vi "AcquireStartCameraAndReferences.vi"(8 "error in (no error)":errorcluster, 9 "?":T2 {"Image Type" items=["Grayscale (U8)", "Grayscale (I16)", "Grayscale (SGL)", "Complex (CSG)", "RGB (U32)", "HSL (U32)", "RGB (U64)", "Grayscale (U16)"]}, 10 "Settings":T4={"Harware Configuration"={"Camera"="cam1", "Frames Per Second"=15, "Simulate Recording"=FALSE, "Simulated Recording Sample"=path "", "Timestamp Method"=enum."Camera Timestamp"}, "Base Recording Path"=path "", "Type Of Recording"="", "Recording Codec"="", "TrackingSettings"={"Max Radius"=0, "Threshold"=160.0, "ROI"={"Left"=0, "Top"=0, "Right"=0, "Bottom"=0, "Rotation"=0.0}}, "Calibration"={"Pixel Width (X)"=1.0, "Pixel Height (Y)"=1.0}, "Broadcast Length"=0} {"Broadcast Length" min=0; "TrackingSettings"."ROI"."Rotation" format="%.2f"; "TrackingSettings"."ROI"."Left" scale=0.0..1024.0; "TrackingSettings"."ROI"."Right" scale=0.0..1024.0; "TrackingSettings"."Threshold" scale=0.0..255.0}) -> (0 "error out":errorcluster, 1 "?":T2 {"Image Type" items=["Grayscale (U8)", "Grayscale (I16)", "Grayscale (SGL)", "Complex (CSG)", "RGB (U32)", "HSL (U32)", "RGB (U64)", "Grayscale (U16)"]})   [LabVIEW 2017, in "ImageAcquisitionLibrary.lvlib"]
uses:
  ImageAcquisitionLibrary.lvlib
  Settings/Settings.ctl
  <vilib>/userdefined/High Color/IMAQdx.ctl
  Tracking/TrackingSettings.ctl
  Settings/Calibration.ctl
  AcquisitionObject.ctl
  <vilib>/vision/Image Controls.llb/IMAQ Image.ctl
  <vilib>/vision/driver/NI_Vision_Acquisition_Software.lvlib
panel:
  out "Image":T1(plugin-control)
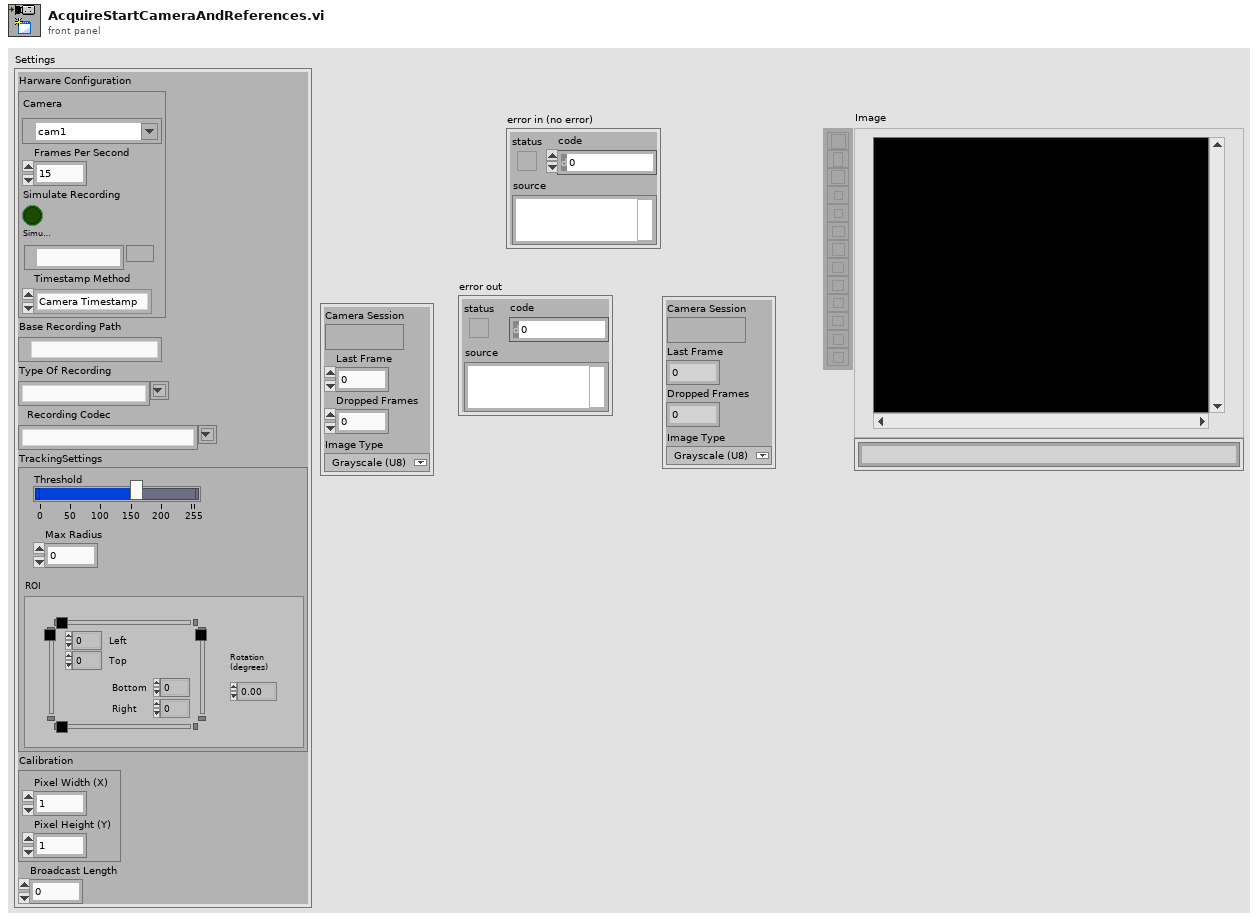
[diagram p1: front panel]
types:
  T1 = typedef "IMAQ Image.ctl" = refnum<image>
  T2 = typedef "ImageAcquisitionLibrary.lvlib/AcquisitionObject.ctl" = cluster{"Camera Session":T1, "Last Frame":u32, "Dropped Frames":u32, "Image Type":T3}
  T3 = typedef "Image Type" = u32
  T4 = typedef "ImageAcquisitionLibrary.lvlib/Settings.ctl" = cluster{"Harware Configuration":cluster{"Camera":T5, "Frames Per Second":u32, "Simulate Recording":bool, "Simulated Recording Sample":path, "Timestamp Method":enum16{"System Timestamp", "Camera Timestamp", "IMAQdx Timestamp"}}, "Base Recording Path":path, "Type Of Recording":string, "Recording Codec":string, "TrackingSettings":T6, "Calibration":T8, "Broadcast Length":i32}
  T5 = typedef "IMAQdx.ctl" = refnum<k21>
  T6 = typedef "ImageAcquisitionLibrary.lvlib/TrackingSettings.ctl" = cluster{"Max Radius":i32, "Threshold":sgl, "ROI":T7}
  T7 = typedef "IMAQ Rectangle" = cluster{"Left":i32, "Top":i32, "Right":i32, "Bottom":i32, "Rotation":dbl}
  T8 = typedef "ImageAcquisitionLibrary.lvlib/Calibration.ctl" = cluster{"Pixel Width (X)":dbl, "Pixel Height (Y)":dbl}
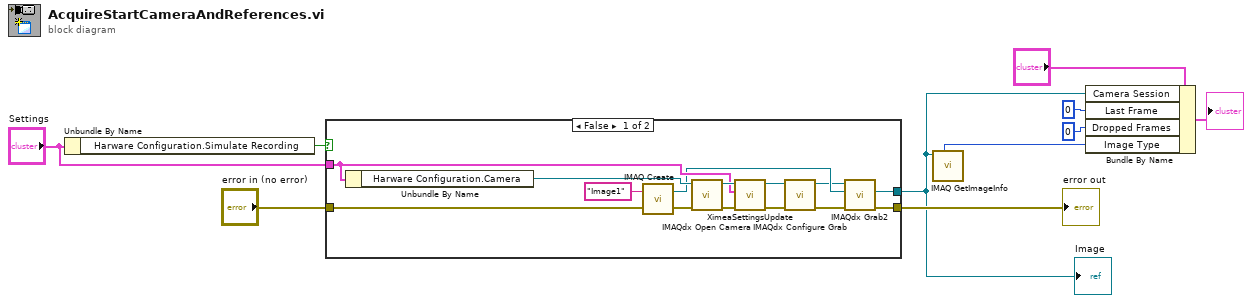
[diagram p0: block diagram]
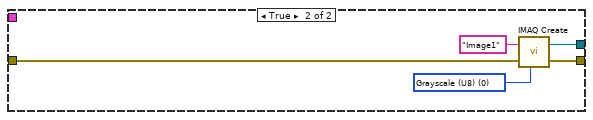
[diagram p2: hidden frame]
diagram:
  n1 = Unbundle By Name("Settings") -> ("Harware Configuration.Simulate Recording"=w9:bool)
  n2 = case shown="False" w9 {
    tunnel: "Settings" -> [w16 _]
    tunnel: "error in (no error)" -> [w23 w27]
    tunnel: [w11 w26] -> w2
    tunnel: [w14 w25] -> w3
    frame False {
      n3 = Unbundle By Name(w16) -> ("Harware Configuration.Camera"=w20:T5)
      n4 = call "IMAQ Create"("Image Name"="Image1", "error in (no error)"=w23) -> ("New Image"=w13:T1, "error out"=w19:errorcluster)  [unwired: 3 in]
      n5 = call <vilib>:"IMAQdx Open Camera.vi"("error in"=w19, "Session In"=w20) -> ("error out"=w21:errorcluster, "Session Out"=w22:T5)  [unwired: 8 in]
      n6 = call "XimeaSettingsUpdate.vi"("error in"=w21, "Cluster"=w16, "Session In"=w22) -> ("error out"=w18:errorcluster, "IMAQdx Session"=w17:T5)  [unwired: 7 in]
      n7 = call <vilib>:"IMAQdx Configure Grab.vi"("error in"=w18, "Session In"=w17) -> ("error out"=w15:errorcluster, "Session Out"=w12:T5)  [unwired: 8 in]
      n8 = call <vilib>:"IMAQdx Grab2.vi"("error in"=w15, "Image In"=w13, "Session In"=w12) -> ("error out"=w14:errorcluster, "Image Out"=w11:T1)  [unwired: 5 in, 2 out]
    }
    frame True {
      w29 = T3 0 items=["Grayscale (U8)", "Grayscale (I16)", "Grayscale (SGL)", "Complex (CSG)", "RGB (U32)", "HSL (U32)", "RGB (U64)", "Grayscale (U16)"] ("Image Type")
      n9 = call "IMAQ Create"("Image Name"="Image1", "Image Type"=w29, "error in (no error)"=w27) -> ("New Image"=w26:T1, "error out"=w25:errorcluster)  [unwired: 2 in]
    }
  }
  "error out" <- w3
  "Image" <- w2
  n10 = call "IMAQ GetImageInfo"("Image"=w2) -> ("Image Type"=w1:T3)  [unwired: 3 in, 7 out]
  n11 = Bundle By Name(cluster="?", "Camera Session"=w2, "Last Frame"=u32 0, "Dropped Frames"=u32 0, "Image Type"=w1) -> (→"?":T2)
